vi "AcquireInpuData.vi"(0 "device ID":refnum<k1>, 1 "key mode":enum16{"RELATIVE", "ABSOLUTE"}(ring)=enum."ABSOLUTE", 5 "error in (no error)":errorcluster) -> (14 "device ID":refnum<k1>, 15 "axis info":T2, 16 "button info":T1, 19 "error out":errorcluster)   [LabVIEW 2011]
doc: "Returns data about the device connected to the computer. Wire data to the <B>device ID</B> input to determine the polymorphic instance to use or manually select the instance."
uses:
  Program Files/National Instruments/LabVIEW 2011/resource/lvinput.dll
panel:
  in  "Input Value":i8[](array[numeric])=[0, 0, 0, 0, 0]
  out "Axis Info":i32[](array[numeric])
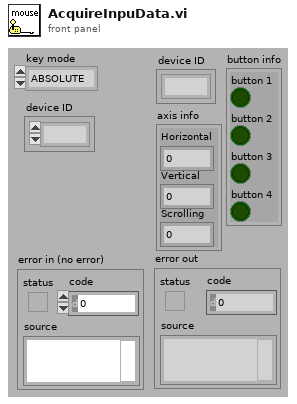
[diagram p1: front panel]
types:
  T1 = cluster{"button 1":bool, "button 2":bool, "button 3":bool, "button 4":bool}
  T2 = cluster{"Horizontal":i32, "Vertical":i32, "Scrolling":i32}
  T3 = cluster{"[0]":bool, "[1]":bool, "[2]":bool, "[3]":bool}
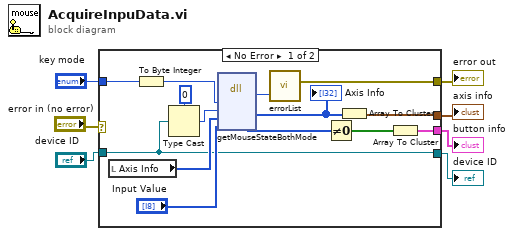
[diagram p0: block diagram]
diagram:
  n1 = case shown="No Error" "error in (no error)" {
    selector: "error in (no error)" -> [_ w22]
    tunnel: [w10 w22] -> w7
    tunnel: [w13 cluster{i32, i32, i32} {0, 0, 0}] -> w5
    tunnel: [w11 cluster{bool, bool, bool, bool} {FALSE, FALSE, FALSE, FALSE}] -> w3
    tunnel: "device ID" -> [w8 w23]
    tunnel: [w8 w23] -> w2
    tunnel: "key mode" -> [w9 _]
    frame No Error {
      n2 = local read "Axis Info"() -> (w18:i32[])
      n3 = To Byte Integer(number=w9) -> (8bit integer=w15:i8)
      n4 = Type Cast(type=0, x=w8) -> (*(type *) &x=w19:i32)
      n5 = dll-call lib="C:/Program Files/National Instruments/LabVIEW 2011/resource/lvinput.*" fn="getMouseStateBothMode"(w15, w19, w18, "Input Value") -> (w21:i32, w14:i32[], w16:i8[])  [unwired: 5 in, 2 out]
      "Axis Info" <- w14
      n6 = call <vilib>:"errorList.vi"("ERROR CODE"=w21) -> ("error in 1 (no error)"=w10:errorcluster)
      n7 = Not Equal To 0?(x=w16) -> (x != 0?=w12:bool[])
      n8 = Array To Cluster(array=w14) -> (cluster=w13:cluster{"[0]":i32, "[1]":i32, "[2]":i32})
      n9 = Array To Cluster(array=w12) -> (cluster=w11:T3)
    }
    frame Error {
    }
  }
  "error out" <- w7
  "axis info" <- w5
  "button info" <- w3
  "device ID" <- w2
